vi "CLIMB SYSTEM.vi"(6 "Numeric":i32, 9 "Boolean 2":bool, 10 "Boolean":bool, 11 "Boolean 3":bool) -> ()   [LabVIEW 2019]
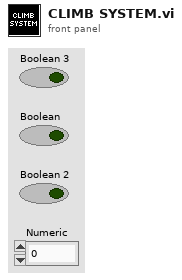
[diagram p1: front panel]
types:
  T1 = typedef "WPI_MotorControlDeviceRef.ctl" = cluster{"DeviceStatus":errorcluster, "Type":T2, "PWM":cluster{"PWM Channel":T3, "DeadBand":T4}, "CAN":cluster{"Device Number":u8, "SetOutput VI Ref":variant, "GetOutput VI Ref":variant, "Enable VI Ref":variant, "Disable VI Ref":variant, "Data":variant}, "Invert":bool, "DIO PWM":cluster{"PWM \"Enable\" Channel":T3, "DIOChannel":T5, "PWM Rate":dbl}}
  T2 = typedef "WPI_MotorControlType.ctl" = enum16{"PWM", "CAN", "DIO PWM"}
  T3 = typedef "FPGA_DIOPWMChannel.ctl" = enum8{"PWM 0", "PWM 1", "PWM 2", "PWM 3", "PWM 4", "PWM 5", "PWM 6", "PWM 7", "PWM 8", "PWM 9", "PWM MXP 0", "PWM MXP 1", "PWM MXP 2", "PWM MXP 3", "PWM MXP 4", "PWM MXP 5", "PWM MXP 6", "PWM MXP 7", "PWM MXP 8", "PWM MXP 9", "Invalid"}
  T4 = typedef "WPI_PWMDeadband.ctl" = cluster{"Name":string, "maxPositivePwm":i32, "minPositivePwm":i32, "centerPwm":i32, "maxNegativePwm":i32, "minNegativePwm":i32, "angularRange":u16}
  T5 = typedef "FPGA_DIOChannel.ctl" = enum8{"DIO 0", "DIO 1", "DIO 2", "DIO 3", "DIO 4", "DIO 5", "DIO 6", "DIO 7", "DIO 8", "DIO 9", "DIO MXP 0", "DIO MXP 1", "DIO MXP 2", "DIO MXP 3", "DIO MXP 4", "DIO MXP 5", "DIO MXP 6", "DIO MXP 7", "DIO MXP 8", "DIO MXP 9", "DIO MXP 10", "DIO MXP 11", "DIO MXP 12", "DIO MXP 13", "DIO MXP 14", "DIO MXP 15", "SPI Port CS1", "SPI Port CS2", "SPI Port CS3", "SPI Port MISO", "SPI Port MOSI", "Invalid"}
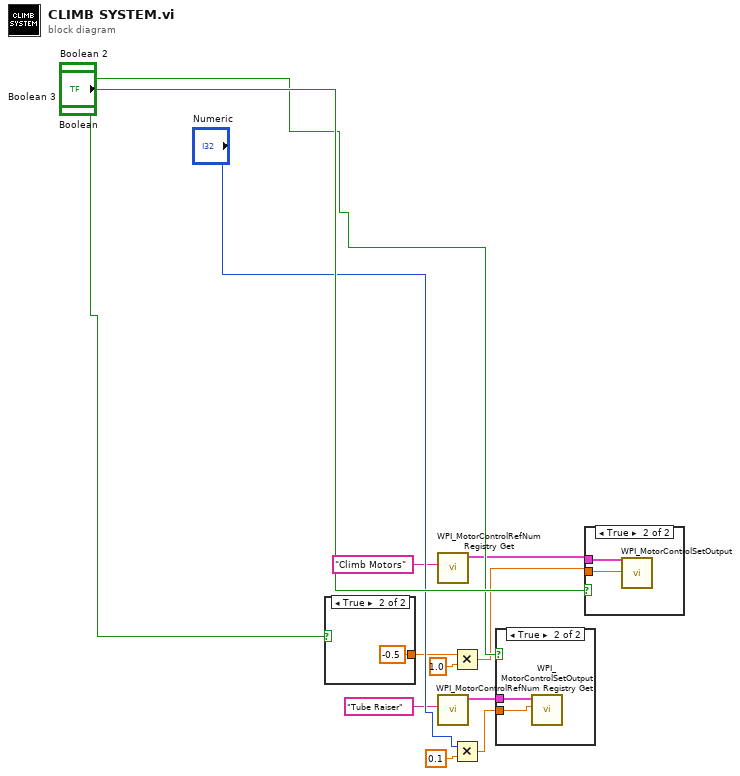
[diagram p0: block diagram]
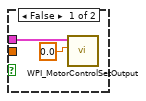
[diagram p2: hidden frame]
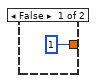
[diagram p3: hidden frame]
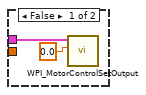
[diagram p4: hidden frame]
diagram:
  n1 = case shown="True" "Boolean 3" {
    tunnel: [1 -0.5] -> w9
    frame False {
    }
    frame True {
    }
  }
  n2 = call <vilib>:"WPI_MotorControlRefNum Registry Get.vi"("refnum name"="Climb Motors") -> ("MotorControlDevRef"=w6:T1)  [unwired: 9 in, 1 out]
  n3 = call <vilib>:"WPI_MotorControlRefNum Registry Get.vi"("refnum name"="Tube Raiser") -> ("MotorControlDevRef"=w2:T1)  [unwired: 9 in, 1 out]
  n4 = Multiply(x=w9, y=1.0 ("Output")) -> (x*y=w8:dbl)
  n5 = Multiply(x="Numeric", y=0.1 ("Output")) -> (x*y=w4:dbl)
  n6 = case shown="True" "Boolean 2" {
    tunnel: w2 -> [w16 w19]
    tunnel: w4 -> [_ w18]
    frame False {
      n7 = call <vilib>:"WPI_MotorControlSetOutput.vi"("Output"=0.0, "MotorControlDevRef"=w16) -> ()  [unwired: 7 in, 3 out]
    }
    frame True {
      n8 = call <vilib>:"WPI_MotorControlSetOutput.vi"("Output"=w18, "MotorControlDevRef"=w19) -> ()  [unwired: 7 in, 3 out]
    }
  }
  n9 = case shown="True" "Boolean" {
    tunnel: w6 -> [w20 w23]
    tunnel: w8 -> [_ w22]
    frame False {
      n10 = call <vilib>:"WPI_MotorControlSetOutput.vi"("Output"=0.0, "MotorControlDevRef"=w20) -> ()  [unwired: 7 in, 3 out]
    }
    frame True {
      n11 = call <vilib>:"WPI_MotorControlSetOutput.vi"("Output"=w22, "MotorControlDevRef"=w23) -> ()  [unwired: 7 in, 3 out]
    }
  }
